vi "Drum Subvi w Notes on Off 2.vi"(5 "Drum Notes On/Off":bool, 8 "Image Dst Out":T1) -> (7 "Red Drum":bool, 9 "Yellow Array":bool[](array[boolean]), 13 "Foot Pedal":bool, 16 "Blue array":bool[](array[boolean]), 17 "Red Array":bool[](array[boolean]), 20 "Green Array":bool[](array[boolean]), 23 "Blue Drum 2":bool, 24 "Yellow Drum":bool, 25 "Green Drum":bool)   [LabVIEW 2009]
uses:
  <vilib>/vision/Image Controls.llb/IMAQ Image.ctl
  <vilib>/Analysis/3filter.llb/Filter Passband Type.ctl
  <vilib>/Analysis/3filter.llb/Butterworth Filter (DBL).vi
  <vilib>/Analysis/NI_AALBase.lvlib
  <vilib>/vision/NI_Vision_Development_Module.lvlib
panel:
  in  "Red Line":T2={"Global Rectangle"=[300, 297, 320, 380], "Contours"=[{"ID"=enum."External", "Type"=2, "Coordinates"=[300, 379, 319, 297]}]} {"Contours"."Type" items=["No Selection", "Point", "Line", "Rectangle", "Oval", "Polygon", "Freehand Region", "Annulus", "Unused2", "Unused3", "Broken Line", "Freehand Line", "Rotated Rectangle"]}
  in  "Blue Line":T2={"Global Rectangle"=[374, 278, 383, 377], "Contours"=[{"ID"=enum."External", "Type"=2, "Coordinates"=[382, 376, 374, 278]}]} {"Contours"."Type" items=["No Selection", "Point", "Line", "Rectangle", "Oval", "Polygon", "Freehand Region", "Annulus", "Unused2", "Unused3", "Broken Line", "Freehand Line", "Rotated Rectangle"]}
  in  "Green Line":T2={"Global Rectangle"=[406, 309, 423, 383], "Contours"=[{"ID"=enum."External", "Type"=2, "Coordinates"=[422, 382, 406, 309]}]} {"Contours"."Type" items=["No Selection", "Point", "Line", "Rectangle", "Oval", "Polygon", "Freehand Region", "Annulus", "Unused2", "Unused3", "Broken Line", "Freehand Line", "Rotated Rectangle"]}
  in  "Yellow Line":T2={"Global Rectangle"=[342, 292, 349, 377], "Contours"=[{"ID"=enum."External", "Type"=2, "Coordinates"=[342, 376, 348, 292]}]} {"Contours"."Type" items=["No Selection", "Point", "Line", "Rectangle", "Oval", "Polygon", "Freehand Region", "Annulus", "Unused2", "Unused3", "Broken Line", "Freehand Line", "Rotated Rectangle"]}
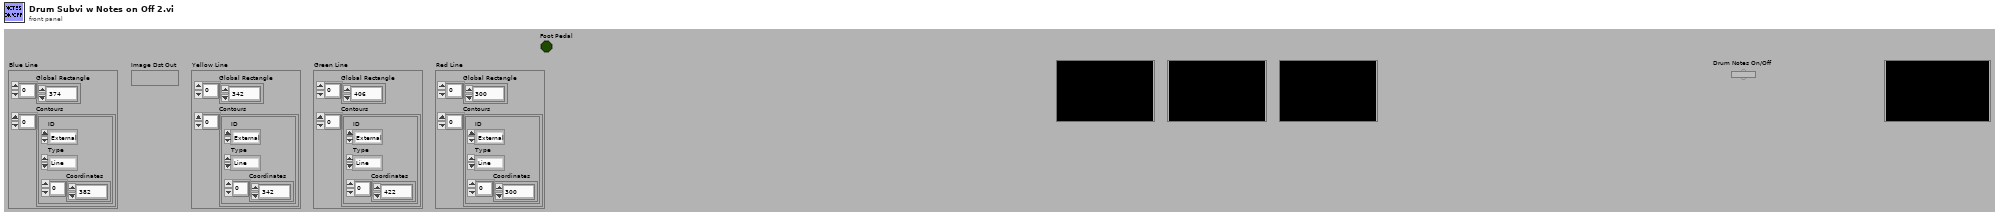
[diagram p1: front panel]
types:
  T1 = typedef "IMAQ Image.ctl" = refnum<image>
  T2 = cluster{"Global Rectangle":i32[], "Contours":cluster{"ID":enum32{"External", "Internal"}, "Type":u32, "Coordinates":i32[]}[]}
  T3 = typedef "NI_AALBase.lvlib/Filter Passband Type.ctl" = enum32{"Lowpass", "Highpass", "Bandpass", "Bandstop"}
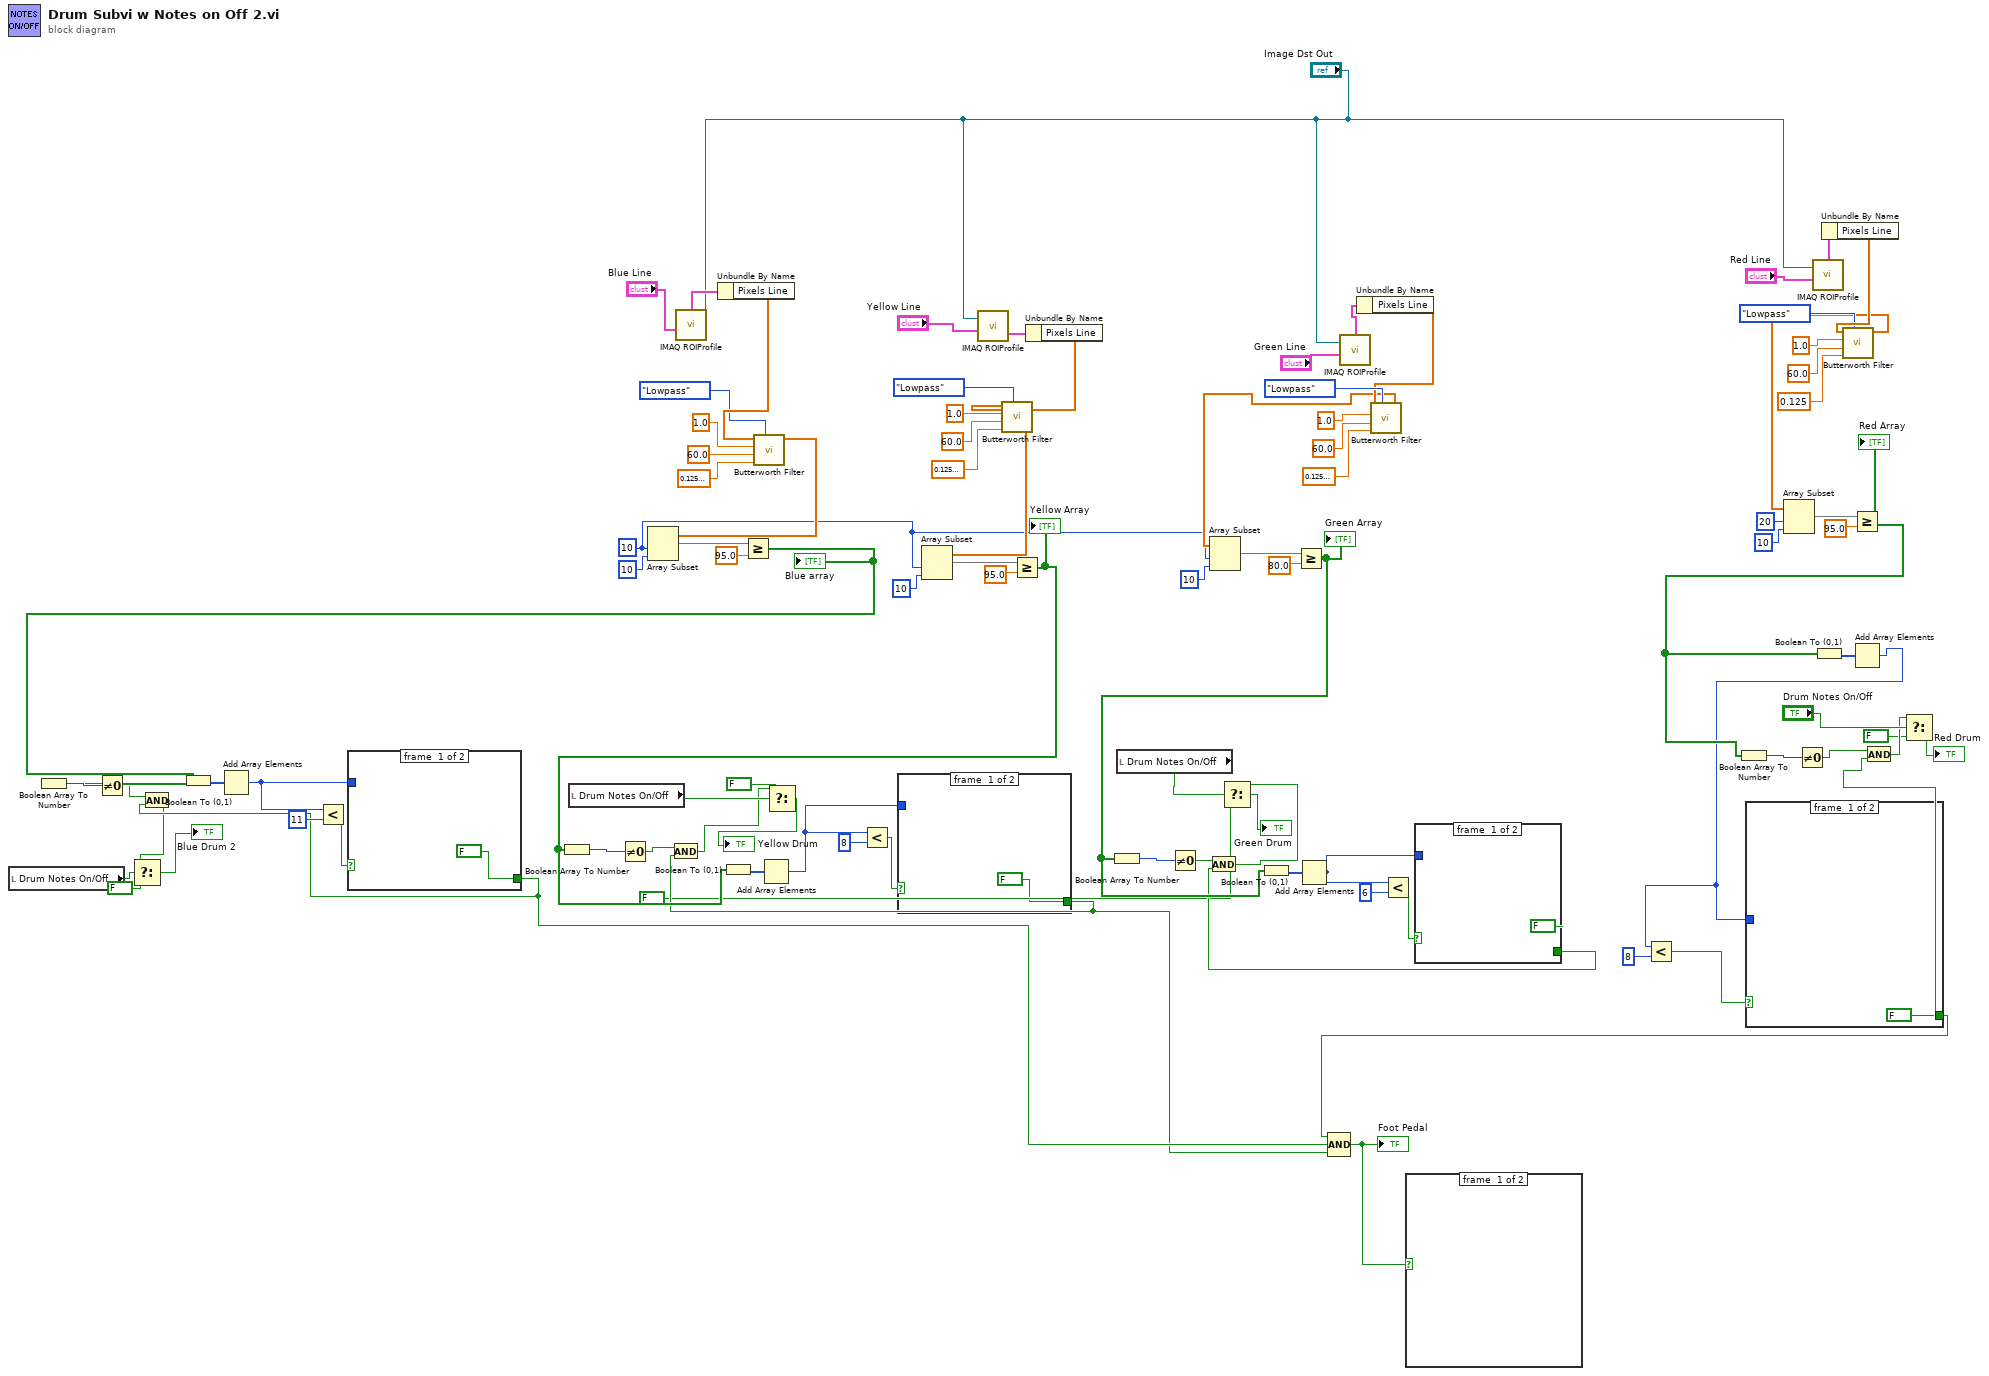
[diagram p0: block diagram]
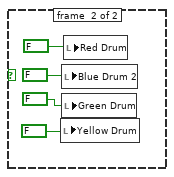
[diagram p2: hidden frame]
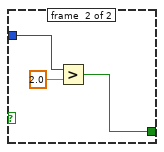
[diagram p3: hidden frame]
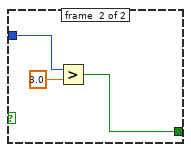
[diagram p4: hidden frame]
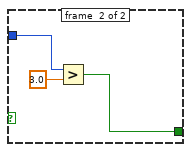
[diagram p5: hidden frame]
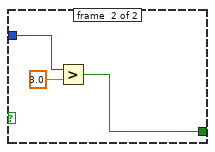
[diagram p6: hidden frame]
diagram:
  w2 = 10 ("index")
  n1 = local read "Drum Notes On/Off"() -> (w18:bool)
  n2 = local read "Drum Notes On/Off"() -> (w19:bool)
  n3 = call "IMAQ ROIProfile"("ROI Descriptor"="Blue Line", "Image"="Image Dst Out") -> ("ROI Graph"=w73:cluster{"x0":sgl, "dx":sgl, "Pixels Line":sgl[]})  [unwired: 1 in, 5 out]
  n4 = Unbundle By Name(w73) -> ("Pixels Line"=w57:sgl[])
  n5 = call-poly <vilib>:"Butterworth Filter.vi"("filter type"=Filter_Passband_Type."Lowpass", "low cutoff freq: fl"=0.12500000000000006 ("low"), "high cutoff freq: fh"=60.0 ("high"), "sampling freq: fs"=1.0 ("sampling"), "X"=w57) -> ("Filtered X"=w83:dbl[])  [unwired: 3 in, 1 out]
  n6 = Array Subset(array=w83, index=w2, length=10) -> (w62:dbl[])
  n7 = Greater Or Equal?(x=w62, y=95.0) -> (x >= y?=w39:bool[])
  "Blue array" <- w39
  n8 = Boolean Array To Number(Boolean array=w39) -> (number=w54:u32)
  n9 = Not Equal To 0?(x=w54) -> (x != 0?=w27:bool)
  n10 = Boolean To (0,1)(Boolean=w39) -> (0, 1=w46:i16[])
  n11 = Add Array Elements(numeric array=w46) -> (sum=w38:i16)
  n12 = Less?(x=w38, y=i16 11) -> (x < y?=w48:bool)
  n13 = case shown="True" w48 {
    tunnel: w38 -> [_ w100]
    tunnel: [FALSE w99] -> w26
    frame #0 {
    }
    frame #1 {
      n14 = Greater?(x=w100, y=3.0) -> (0:w99:bool)
    }
  }
  n15 = And(x=w27, y=w26) -> (x .and. y?=w17:bool)
  n16 = Select(t=w17, s=w18, f=FALSE) -> (s? t:f=→"Blue Drum 2":bool)
  n17 = call "IMAQ ROIProfile"("ROI Descriptor"="Yellow Line", "Image"="Image Dst Out") -> ("ROI Graph"=w70:cluster{"x0":sgl, "dx":sgl, "Pixels Line":sgl[]})  [unwired: 1 in, 5 out]
  n18 = Unbundle By Name(w70) -> ("Pixels Line"=w67:sgl[])
  n19 = call-poly <vilib>:"Butterworth Filter.vi"("filter type"=Filter_Passband_Type."Lowpass", "low cutoff freq: fl"=0.12500000000000006 ("low  2"), "high cutoff freq: fh"=60.0 ("high 2"), "sampling freq: fs"=1.0 ("sampling 2"), "X"=w67) -> ("Filtered X"=w71:dbl[])  [unwired: 3 in, 1 out]
  n20 = Array Subset(array=w71, index=w2, length=10) -> (w64:dbl[])
  n21 = Greater Or Equal?(x=w64, y=95.0) -> (x >= y?=w41:bool[])
  "Yellow Array" <- w41
  n22 = Boolean Array To Number(Boolean array=w41) -> (number=w53:u32)
  n23 = Not Equal To 0?(x=w53) -> (x != 0?=w29:bool)
  n24 = Boolean To (0,1)(Boolean=w41) -> (0, 1=w45:i16[])
  n25 = Add Array Elements(numeric array=w45) -> (sum=w40:i16)
  n26 = Less?(x=w40, y=i16 8) -> (x < y?=w37:bool)
  n27 = case shown="True" w37 {
    tunnel: w40 -> [_ w104]
    tunnel: [FALSE w103] -> w25
    frame #0 {
    }
    frame #1 {
      n28 = Greater?(x=w104, y=3.0) -> (0:w103:bool)
    }
  }
  n29 = And(x=w29, y=w25) -> (x .and. y?=w13:bool)
  n30 = Select(t=w13, s=w19, f=FALSE) -> (s? t:f=→"Yellow Drum":bool)
  n31 = local read "Drum Notes On/Off"() -> (w20:bool)
  n32 = call "IMAQ ROIProfile"("ROI Descriptor"="Green Line", "Image"="Image Dst Out") -> ("ROI Graph"=w74:cluster{"x0":sgl, "dx":sgl, "Pixels Line":sgl[]})  [unwired: 1 in, 5 out]
  n33 = Unbundle By Name(w74) -> ("Pixels Line"=w77:sgl[])
  n34 = call-poly <vilib>:"Butterworth Filter.vi"("filter type"=Filter_Passband_Type."Lowpass", "low cutoff freq: fl"=0.12500000000000006 ("low  3"), "high cutoff freq: fh"=60.0 ("high 3"), "sampling freq: fs"=1.0 ("sampling 3"), "X"=w77) -> ("Filtered X"=w4:dbl[])  [unwired: 3 in, 1 out]
  n35 = Array Subset(array=w4, index=w2, length=10) -> (w80:dbl[])
  n36 = Greater Or Equal?(x=w80, y=80.0) -> (x >= y?=w43:bool[])
  "Green Array" <- w43
  n37 = Boolean Array To Number(Boolean array=w43) -> (number=w52:u32)
  n38 = Not Equal To 0?(x=w52) -> (x != 0?=w28:bool)
  n39 = Boolean To (0,1)(Boolean=w43) -> (0, 1=w44:i16[])
  n40 = Add Array Elements(numeric array=w44) -> (sum=w42:i16)
  n41 = Less?(x=w42, y=i16 6) -> (x < y?=w34:bool)
  n42 = case shown="True" w34 {
    tunnel: w42 -> [_ w108]
    tunnel: [FALSE w107] -> w24
    frame #0 {
    }
    frame #1 {
      n43 = Greater?(x=w108, y=2.0) -> (0:w107:bool)
    }
  }
  n44 = And(x=w28, y=w24) -> (x .and. y?=w7:bool)
  n45 = Select(t=w7, s=w20, f=FALSE) -> (s? t:f=→"Green Drum":bool)
  n46 = call "IMAQ ROIProfile"("ROI Descriptor"="Red Line", "Image"="Image Dst Out") -> ("ROI Graph"=w93:cluster{"x0":sgl, "dx":sgl, "Pixels Line":sgl[]})  [unwired: 1 in, 5 out]
  n47 = Unbundle By Name(w93) -> ("Pixels Line"=w90:sgl[])
  n48 = call-poly <vilib>:"Butterworth Filter.vi"("filter type"=Filter_Passband_Type."Lowpass", "low cutoff freq: fl"=0.125 ("low  4"), "high cutoff freq: fh"=60.0 ("high 4"), "sampling freq: fs"=1.0 ("sampling 4"), "X"=w90) -> ("Filtered X"=w22:dbl[])  [unwired: 3 in, 1 out]
  n49 = Array Subset(array=w22, index=20, length=10) -> (w87:dbl[])
  n50 = Greater Or Equal?(x=w87, y=95.0) -> (x >= y?=w31:bool[])
  "Red Array" <- w31
  n51 = Boolean Array To Number(Boolean array=w31) -> (number=w32:u32)
  n52 = Not Equal To 0?(x=w32) -> (x != 0?=w30:bool)
  n53 = Boolean To (0,1)(Boolean=w31) -> (0, 1=w51:i16[])
  n54 = Add Array Elements(numeric array=w51) -> (sum=w3:i16)
  n55 = Less?(x=w3, y=i16 8) -> (x < y?=w49:bool)
  n56 = case shown="True" w49 {
    tunnel: w3 -> [_ w111]
    tunnel: [FALSE w110] -> w33
    frame #0 {
    }
    frame #1 {
      n57 = Greater?(x=w111, y=3.0) -> (0:w110:bool)
    }
  }
  n58 = Compound Arithmetic op=AND(w33, w26, w25) -> (w23:bool)
  "Foot Pedal" <- w23
  n59 = case shown="False" w23 {
    frame #0 {
    }
    frame #1 {
      n60 = local write "Yellow Drum"(FALSE) -> ()
      n61 = local write "Blue Drum 2"(FALSE) -> ()
      n62 = local write "Green Drum"(FALSE) -> ()
      n63 = local write "Red Drum"(FALSE) -> ()
    }
  }
  n64 = And(x=w30, y=w33) -> (x .and. y?=w10:bool)
  n65 = Select(t=w10, s="Drum Notes On/Off", f=FALSE) -> (s? t:f=→"Red Drum":bool)
